vi "Filter Signal.vi"(11 "PASS DC 12V":waveform(dbl)[](graph)=[{"t0"=timestamp(0 s since 1904-01-01), "dt"=2.5e-06, "Y"=array[250000 elements]}, {"t0"=timestamp(0 s since 1904-01-01), "dt"=2.5e-06, "Y"=array[250000 elements]}, {"t0"=timestamp(0 s since 1904-01-01), "dt"=2.5e-06, "Y"=array[250000 elements]}]) -> (1 "Raw":waveform(dbl)(graph), 2 "Filter":waveform(dbl)(graph), 3 "Filter + Smooth":waveform(dbl)(graph))   [LabVIEW 2019]
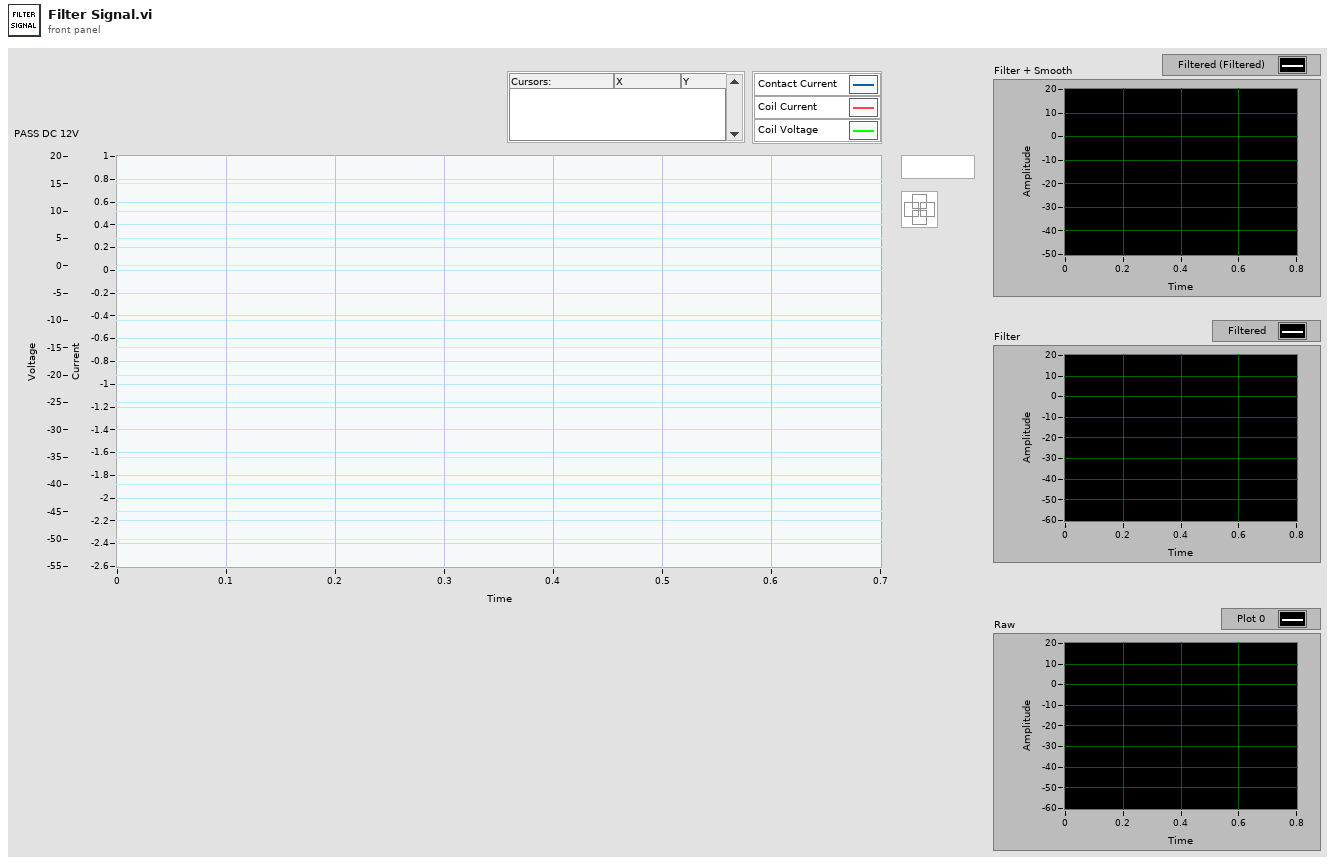
[diagram p1: front panel]
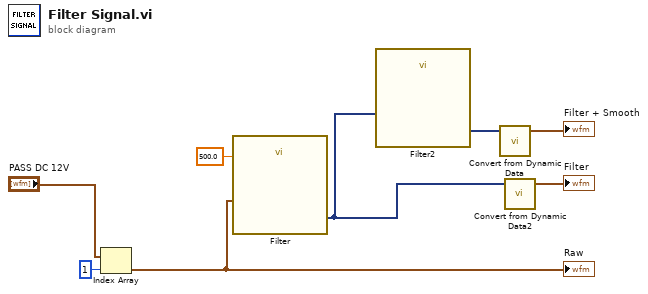
[diagram p0: block diagram]
diagram:
  n1 = Index Array(array="PASS DC 12V", index=1) -> (element=w2:waveform(dbl))
  "Raw" <- w2
  n2 = call "Filter"("Lower Cut-Off"=500.0, "Signal"=w2) -> ("Filtered Signal"=w7:dynamicdata)  [unwired: 8 in, 1 out]
  n3 = call "Filter2"("Signal"=w7) -> ("Filtered Signal"=w5:dynamicdata)  [unwired: 9 in, 1 out]
  n4 = call "Convert from Dynamic Data"("Dynamic Data Type"=w5) -> ("Waveform"=→"Filter + Smooth":waveform(dbl))  [unwired: 3 in]
  n5 = call "Convert from Dynamic Data2"("Dynamic Data Type"=w7) -> ("Waveform"=→"Filter":waveform(dbl))  [unwired: 3 in]
